vi "Close.vi"(8 "error in (no error)":errorcluster, 11 "DB_API.lvclass 2":refnum<class "DB_API.lvclass">) -> (0 "error out":errorcluster)   [LabVIEW 2024, in "DB_API.lvclass"]
uses:
  DB_API.lvclass
  DB_API.lvclass/DB_API.ctl
  <vilib>/httpClient/LabVIEWHTTPClient.lvlib
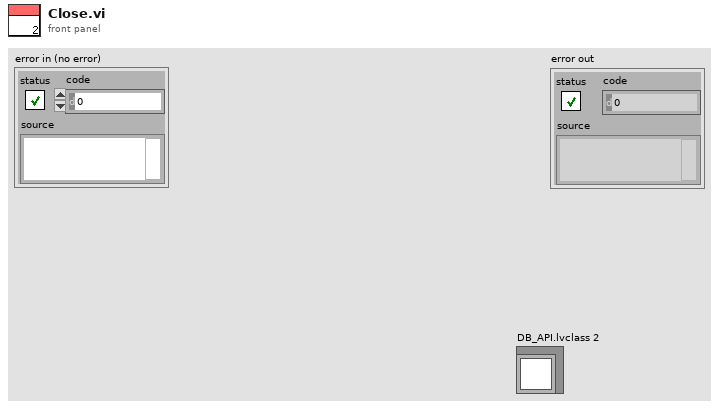
[diagram p1: front panel]
types:
  T1 = typedef "LabVIEWHTTPClient.lvlib/ClientHandle.ctl" = refnum<k1>
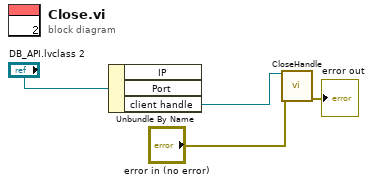
[diagram p0: block diagram]
diagram:
  n1 = Unbundle By Name("DB_API.lvclass 2") -> ("client handle"=w3:T1)  [unwired: 2 out]
  n2 = call <vilib>:"CloseHandle.vi"("client handle"=w3, "error in (no error)"="error in (no error)") -> ("error out"=→"error out":errorcluster)  [unwired: 13 in]
